vi "Configure Continuous Acquisition.vi"(8 "error in (no error)":errorcluster, 9 "Auto Trigger Enabled (T: Normal)":bool=TRUE, 10 "Continuous Acquisition Mode (T: On)":bool=TRUE, 11 "VISA resource name":refnum<visa-resource-name>) -> (0 "error out":errorcluster, 3 "VISA resource name out":refnum<visa-resource-name>)   [LabVIEW 2013, in "LeCroy Wave Series.lvlib"]
doc: "Configures the instrument to run continuously or to stop after a single configured acquisition.\n\nNote:\n(1) This setting does not occur until the <B>Initiate</B> or <B>Read Waveform</B> VI is called.\n(2) Performing an Autosetup, will put the instrument in continuous acquisition mode."
uses:
  LeCroy Wave Series.lvlib
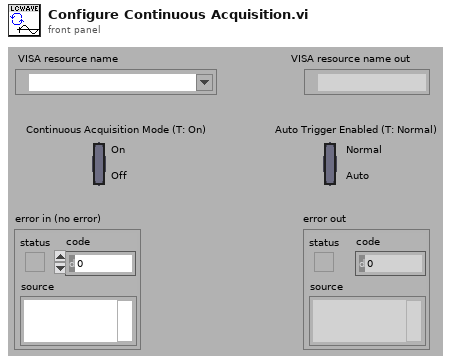
[diagram p1: front panel]
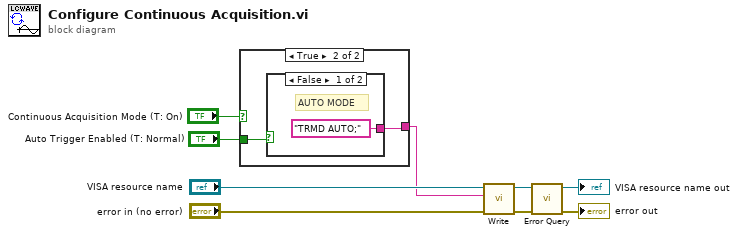
[diagram p0: block diagram]
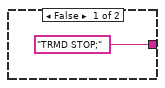
[diagram p2: hidden frame]
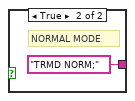
[diagram p3: hidden frame]
diagram:
  n1 = case shown="True" "Continuous Acquisition Mode (T: On)" {
    tunnel: ["TRMD STOP;" w11] -> w2
    tunnel: "Auto Trigger Enabled (T: Normal)" -> [_ w12]
    frame False {
    }
    frame True {
      n2 = case shown="False" w12 {
        tunnel: ["TRMD AUTO;" "TRMD NORM;"] -> w11
        frame False {
          # "AUTO MODE"
        }
        frame True {
          # "NORMAL MODE"
        }
      }
    }
  }
  n3 = call "Write.vi"("error in (no error)"="error in (no error)", "Write Buffer"=w2, "VISA resource name"="VISA resource name") -> ("error out"=w5:errorcluster, "VISA resource name out"=w6:refnum<visa-resource-name>)  [unwired: 6 in, 1 out]
  n4 = call "Error Query.vi"("error in (no error)"=w5, "VISA resource name"=w6) -> ("error out"=→"error out":errorcluster, "VISA resource name out"=→"VISA resource name out":refnum<visa-resource-name>)  [unwired: 6 in, 2 out]
